vi "OAT Recreate Speed Profile for Resample.vi"(5 "lags":i32, 7 "init/continue (init:T)":bool, 8 "output length":i32=1, 9 "decimation factor":i32=1, 10 "sample / rev":dbl=1.0 format="%.2f", 11 "time stamps in":dbl[](array[numeric]) format="%.2f") -> (3 "speed profile":T1 {"speed [RPM]" format="%.2f"; "time [s]" format="%.2f"})   [LabVIEW 2017, in "SoundVib_Resampling.lvlib"]
uses:
  <vilib>/addons/Sound and Vibration/Order Analysis/Resample Order Tracking/SoundVib_Resampling.lvlib
  <vilib>/addons/Sound and Vibration/Order Analysis/Tach Process/SubVIs/speed profile.ctl
  <vilib>/Analysis/2dsp.llb/Decimate (continuous, DBL).vi
  <vilib>/Analysis/NI_AALPro.lvlib
  <vilib>/addons/Sound and Vibration/Order Analysis/Tach Process/SoundVib_TachProcess.lvlib
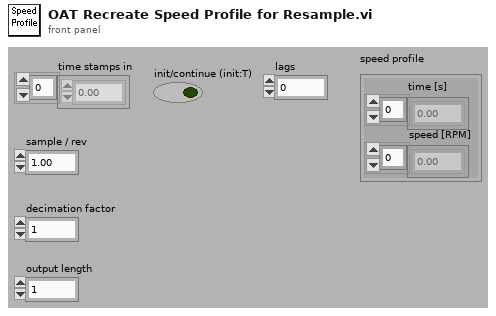
[diagram p1: front panel]
types:
  T1 = typedef "SoundVib_TachProcess.lvlib/speed profile.ctl" = cluster{"time [s]":dbl[], "speed [RPM]":dbl[]}
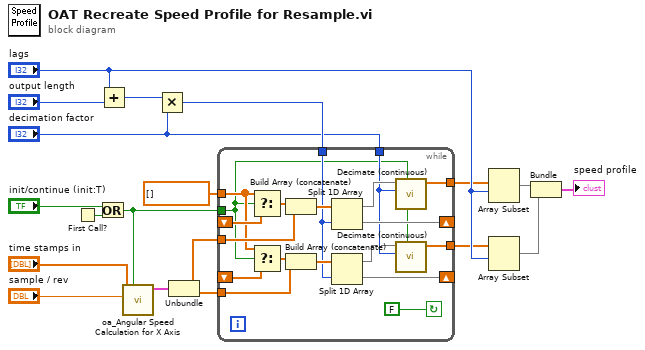
[diagram p0: block diagram]
diagram:
  n1 = First Call?() -> (First Call?: T/F=w19:bool)
  n2 = Or(x="init/continue (init:T)", y=w19) -> (x .or. y?=w9:bool)
  n3 = Add(x="lags", y="output length") -> (x+y=w10:i32)
  n4 = call <vilib>:"oa_Angular Speed Calculation for X Axis.vi"("reset? (True)"=w9, "pulse/revolution (1)"="sample / rev", "pulse positions [s]"="time stamps in") -> ("speed profile"=w1:T1)  [unwired: 7 in, 1 out]
  n5 = Multiply(x=w10, y="decimation factor") -> (x*y=w17:i32)
  n6 = Unbundle(w1) -> ("time [s]"=w5:dbl[], "speed [RPM]"=w4:dbl[])
  n7 = while {
    tunnel: w9 -> [w20]
    shift-right: [w35] -> _
    shift-left: _ -> [w38]
    tunnel: dbl[] [] ("time stamps in") -> [w28]
    tunnel: w5 -> [w36]
    tunnel: w17 -> [w26]
    tunnel: "decimation factor" -> [w22]
    tunnel: [w33] -> w3
    shift-right: [w25] -> _
    shift-left: _ -> [w24]
    tunnel: w4 -> [w27]
    tunnel: [w23] -> w2
    stop <- FALSE continue-if-true
    n8 = Select(t=w28, s=w20, f=w38) -> (s? t:f=w37:dbl[])
    n9 = Select(t=w28, s=w20, f=w24) -> (s? t:f=w29:dbl[])
    n10 = Build Array (concatenate)(w37, w36) -> (w31:dbl[])
    n11 = Build Array (concatenate)(w29, w27) -> (w30:dbl[])
    n12 = Split 1D Array(array=w31, index=w26) -> (first subarray=w32:dbl[], second subarray=w35:dbl[])
    n13 = Split 1D Array(array=w30, index=w26) -> (first subarray=w21:dbl[], second subarray=w25:dbl[])
    n14 = call-poly <vilib>:"Decimate (continuous).vi"("reset"=w20, "decimating factor"=w22, "X"=w32) -> ("Decimated Array"=w33:dbl[])  [unwired: 7 in, 1 out]
    n15 = call-poly <vilib>:"Decimate (continuous).vi"("reset"=w20, "decimating factor"=w22, "X"=w21) -> ("Decimated Array"=w23:dbl[])  [unwired: 7 in, 1 out]
  }
  n16 = Array Subset(array=w3, index="lags") -> (w16:dbl[])  [unwired: 1 in]
  n17 = Array Subset(array=w2, index="lags") -> (w15:dbl[])  [unwired: 1 in]
  n18 = Bundle(w16, w15) -> (→"speed profile":cluster{dbl[], dbl[]})  [unwired: 1 in]
